vi "Error Query.vi"(8 "error in (no error)":errorcluster, 11 "VISA resource name":refnum<visa-resource-name>) -> (0 "error out":errorcluster, 1 "Error Message":string, 2 "Error Code":i32, 3 "VISA resource name out":refnum<visa-resource-name>)   [LabVIEW 2012, in "Micos_uic.lvlib"]
doc: "Queries the instrument for any errors in the instrument's error queue. It will continue to read errors until all errors have been read from the instrument. Any errors will be returned in the <B>error out</B> control.\n\n<B>Note:</B>\nThis VI is called automatically by most driver VIs so it is not usually necessary to call this in an application."
uses:
  <instrlib>/Micos_uic/Micos_uic.lvlib
panel:
  # "EDIT: Note: The Error Query VI is included as a subVI in all driver VIs except low-level API VIs. If the instrument does not support error query, then remove the VI and remove subVI calls in each instrument driver VI that calls it."
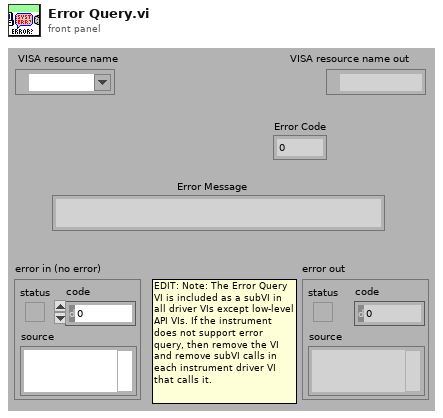
[diagram p1: front panel]
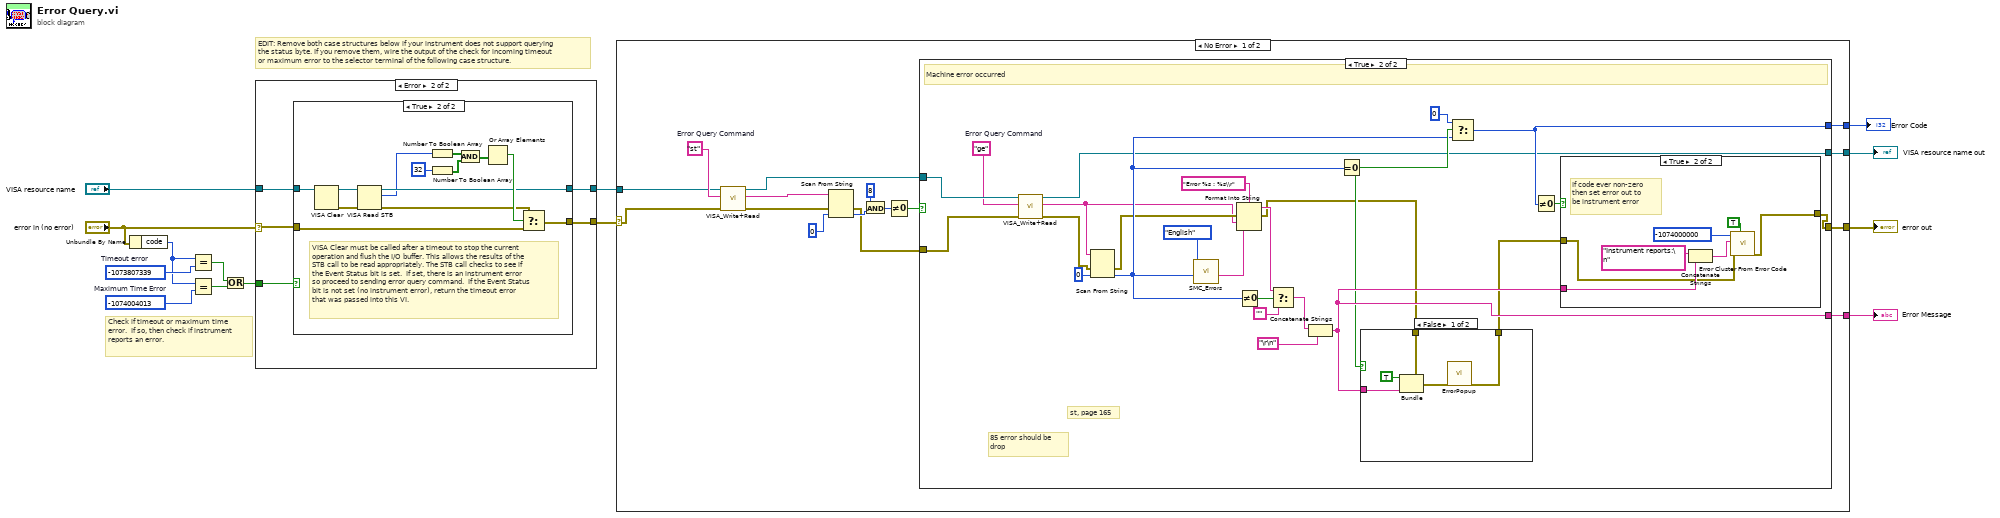
[diagram p0: block diagram]
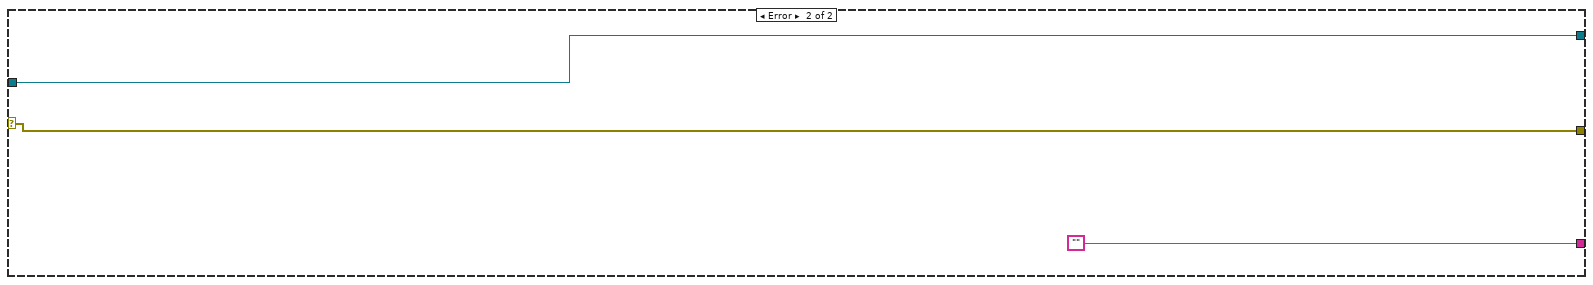
[diagram p7: hidden frame]
diagram:
  w6 = -1074004013  # Maximum Time Error
  w8 = -1073807339  # Timeout error
  # "Check if timeout or maximum time error.  If so, then check if instrument reports an error."
  # "EDIT: Remove both case structures below if your instrument does not support querying the status byte. If you remove them, wire the output of the check for incoming timeout or maximum error to the selector terminal of the following case structure."
  n1 = Unbundle By Name("error in (no error)") -> ("code"=w7:i32)
  n2 = Equal?(x=w7, y=w8) -> (x = y?=w4:bool)
  n3 = Equal?(x=w7, y=w6) -> (x = y?=w5:bool)
  n4 = Or(x=w4, y=w5) -> (x .or. y?=w3:bool)
  n5 = case shown="Error" "error in (no error)" {
    selector: "error in (no error)" -> [w15 w19]
    tunnel: "VISA resource name" -> [w16 w21]
    tunnel: [w16 w20] -> w10
    tunnel: [w15 w18] -> w11
    tunnel: w3 -> [_ w17]
    frame No Error {
    }
    frame Error {
      n6 = case shown="True" w17 {
        tunnel: w21 -> [w23 w29]
        tunnel: [w23 w26] -> w20
        tunnel: w19 -> [w22 w32]
        tunnel: [w22 w31] -> w18
        frame False {
          # "Error code not a timeout, so best to pass on to user."
        }
        frame True {
          # "VISA Clear must be called after a timeout to stop the current operation and flush the I/O buffer. This allows the results of the  STB call to be read appropriately. The STB call checks to see if the Event Status bit is set.  If set, there is an instrument error so proceed to sending error query command.  If the Event Status bit is not set (no instrument error), return the timeout error that was passed into this VI."
          n7 = VISA Clear(VISA resource name=w29) -> (VISA resource name out=w28:refnum<visa-resource-name>, error out=w27:errorcluster)  [unwired: 1 in]
          n8 = VISA Read STB(8:w27, 11:w28) -> (0:w25:errorcluster, 2:w24:u16, 3:w26:refnum<visa-resource-name>)
          n9 = Number To Boolean Array(number=w24) -> (Boolean array=w33:bool[])
          n10 = Number To Boolean Array(number=32) -> (Boolean array=w35:bool[])
          n11 = And(x=w33, y=w35) -> (x .and. y?=w34:bool[])
          n12 = Or Array Elements(Boolean array=w34) -> (logical OR=w30:bool)
          n13 = Select(t=w25, s=w30, f=w32) -> (s? t:f=w31:errorcluster)
        }
      }
    }
  }
  n14 = case shown="No Error" w11 {
    selector: w11 -> [w39 w94]
    tunnel: [w52 w96] -> w14
    tunnel: w10 -> [w41 w96]
    tunnel: [w51 w94] -> w13
    tunnel: [w50 ""] -> w12
    tunnel: [w44 _] -> w1
    frame No Error {
      w42 = "st"  # Error Query Command
      n15 = call <instrlib>:"VISA_Write+Read.vi"("error in (no error)"=w39, "Write Buffer"=w42, "VISA resource name"=w41) -> ("error out"=w38:errorcluster, "readout"=w40:string, "VISA resource name out"=w37:refnum<visa-resource-name>)  [unwired: 6 in]
      n16 = Scan From String(input string=w40, error in=w38, default 1=0) -> (error out=w43:errorcluster, output 1=w47:i32)  [unwired: 2 in, 2 out]
      n17 = And(x=8, y=w47) -> (x .and. y?=w46:i32)
      n18 = Not Equal To 0?(x=w46) -> (x != 0?=w45:bool)
      n19 = case shown="True" w45 {
        tunnel: [w53 w56] -> w52
        tunnel: [w54 w77] -> w51
        tunnel: [_ w76] -> w50
        tunnel: w43 -> [w54 w58]
        tunnel: w37 -> [w53 w60]
        tunnel: [_ w62] -> w44
        frame False {
        }
        frame True {
          w59 = "ge"  # Error Query Command
          # "st, page 165"
          # "85 error should be \ndrop"
          # "Machine error occurred"
          n20 = call <instrlib>:"VISA_Write+Read.vi"("error in (no error)"=w58, "Write Buffer"=w59, "VISA resource name"=w60) -> ("error out"=w57:errorcluster, "readout"=w55:string, "VISA resource name out"=w56:refnum<visa-resource-name>)  [unwired: 6 in]
          n21 = Scan From String(input string=w55, error in=w57, default 1=0) -> (error out=w61:errorcluster, output 1=w63:i32)  [unwired: 2 in, 2 out]
          n22 = call <instrlib>:"SMC_Errors.vi"("Error Code"=w63, "Language"=enum16{"Deutsch", "English"}."English") -> ("Answer"=w70:string)  [unwired: 9 in]
          n23 = Format Into String(format string="Error %s : %s\\r", error in=w61, w55, w70) -> (resulting string=w71:string, error out=w65:errorcluster)  [unwired: 1 in]
          n24 = Not Equal To 0?(x=w63) -> (x != 0?=w68:bool)
          n25 = Select(t=w71, s=w68, f="") -> (s? t:f=w64:string)
          n26 = Concatenate Strings(w64, "\r\n") -> (w76:string)
          n27 = Equal To 0?(x=w63) -> (x = 0?=w73:bool)
          n28 = case shown="False" w73 {
            tunnel: w76 -> [w84 _]
            tunnel: w65 -> [w83 w85]
            tunnel: [w80 w85] -> w75
            frame False {
              n29 = Bundle(cluster=w83, "status"=TRUE, "source"=w84) -> (w81:errorcluster)  [unwired: 1 in]
              n30 = call <instrlib>:"ErrorPopup.vi"("error in (no error)"=w81) -> ("error out"=w80:errorcluster)  [unwired: 10 in]
            }
            frame True {
            }
          }
          n31 = Select(t=0, s=w73, f=w63) -> (s? t:f=w62:i32)
          n32 = Not Equal To 0?(x=w62) -> (x != 0?=w78:bool)
          n33 = case shown="True" w78 {
            tunnel: w76 -> [_ w92]
            tunnel: [w86 w88] -> w77
            tunnel: w75 -> [w86 w87]
            frame False {
            }
            frame True {
              # "If code ever non-zero\nthen set error out to\nbe instrument error"
              n34 = Concatenate Strings("Instrument reports:\n" ("Source"), w92) -> (w89:string)
              n35 = call <vilib>:"Error Cluster From Error Code.vi"("show call chain? (False)"=TRUE, "error in (no error)"=w87, "error message (\"\")"=w89, "error code (0)"=-1074000000 ("Code")) -> ("error out"=w88:errorcluster)  [unwired: 5 in]
            }
          }
        }
      }
    }
    frame Error {
    }
  }
  "VISA resource name out" <- w14
  "error out" <- w13
  "Error Message" <- w12
  "Error Code" <- w1
